vi "createTcpServer.vi"(8 "error in (no error)":errorcluster, 11 "FactoryTcpServer in":refnum<class "FactoryTcpServer.lvclass">) -> (0 "error out":errorcluster, 2 "TcpServer out":refnum<class "TcpServer.lvclass">, 3 "FactoryTcpServer out":refnum<class "FactoryTcpServer.lvclass">)   [LabVIEW 2018, in "FactoryTcpServer.lvclass"]
doc: "Create a new instance of TcpServer class."
uses:
  FactoryTcpServer.lvclass
  TcpServer/TcpServer.lvclass
  TcpServerBase/TcpServerBase.lvclass
  TcpServerCmd/TcpServerCmd.lvclass
  home/pcortes/Documents/github/ts_labview_tcp_json/src/TcpServerBase/TcpServerBase.lvclass
  TcpServerTel/TcpServerTel.lvclass
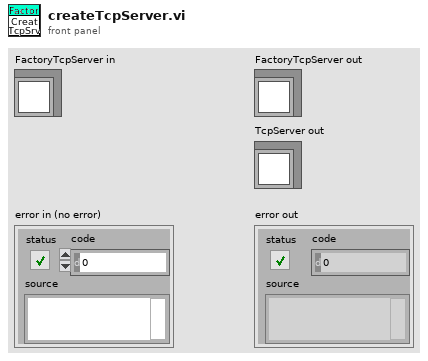
[diagram p1: front panel]
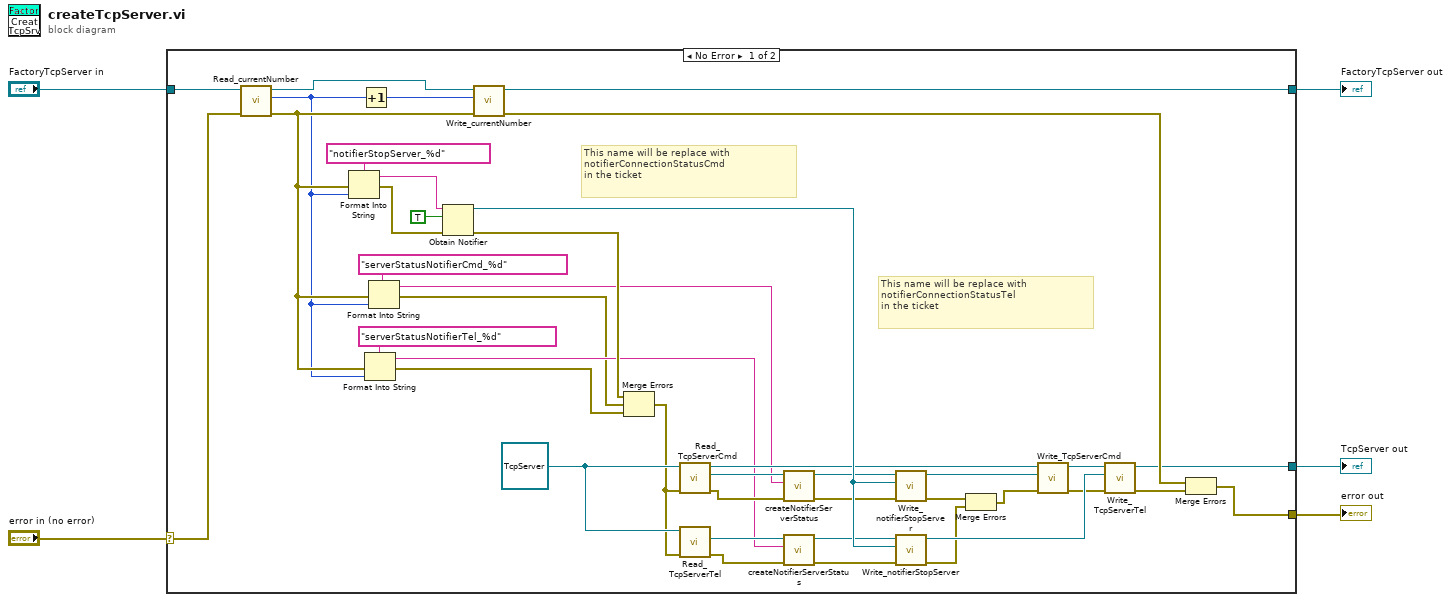
[diagram p0: block diagram]
diagram:
  n1 = case shown="No Error" "error in (no error)" {
    selector: "error in (no error)" -> [w45 w48]
    tunnel: "FactoryTcpServer in" -> [w46 w47]
    tunnel: [w25 w48] -> w3
    tunnel: [w41 w47] -> w2
    tunnel: [w30 _] -> w1
    frame No Error {
      w38 = refnum<class "TcpServer.lvclass"> refnum ("TcpServer.lvclass")
      # "This name will be replace with \nnotifierConnectionStatusTel\nin the ticket"
      # "This name will be replace with \nnotifierConnectionStatusCmd \nin the ticket"
      n2 = call "Read_currentNumber.vi"("error in (no error)"=w45, "FactoryTcpServer in"=w46) -> ("error out"=w20:errorcluster, "currentNumber"=w19:i32, "FactoryTcpServer out"=w42:refnum<class "FactoryTcpServer.lvclass">)  [unwired: 7 in]
      n3 = Format Into String(format string="notifierStopServer_%d", error in=w20, w19) -> (resulting string=w39:string, error out=w23:errorcluster)  [unwired: 1 in]
      n4 = Increment(x=w19) -> (x+1=w44:i32)
      n5 = Format Into String(format string="serverStatusNotifierTel_%d", error in=w20, w19) -> (resulting string=w8:string, error out=w6:errorcluster)  [unwired: 1 in]
      n6 = Format Into String(format string="serverStatusNotifierCmd_%d", error in=w20, w19) -> (resulting string=w10:string, error out=w7:errorcluster)  [unwired: 1 in]
      n7 = Obtain Notifier(name (unnamed)=w39, notification data type=TRUE, error in (no error)=w23) -> (notifier out=w36:refnum<notifier>, error out=w11:errorcluster)  [unwired: 1 in, 1 out]
      n8 = call "Write_currentNumber.vi"("error in (no error)"=w20, "currentNumber"=w44, "FactoryTcpServer in"=w42) -> ("error out"=w43:errorcluster, "FactoryTcpServer out"=w41:refnum<class "FactoryTcpServer.lvclass">)  [unwired: 7 in]
      n9 = Merge Errors(w11, w7, w6) -> (w12:errorcluster)
      n10 = call "Read_TcpServerCmd.vi"("error in (no error)"=w12, "TcpServer in"=w38) -> ("error out"=w9:errorcluster, "TcpServerCmd.lvclass"=w18:refnum<class "TcpServerCmd.lvclass">, "TcpServer out"=w34:refnum<class "TcpServer.lvclass">)  [unwired: 7 in]
      n11 = call "Read_TcpServerTel.vi"("error in (no error)"=w12, "TcpServer in"=w38) -> ("error out"=w29:errorcluster, "TcpServerTel.lvclass"=w15:refnum<class "TcpServerTel.lvclass">)  [unwired: 7 in, 1 out]
      n12 = call "createNotifierServerStatus.vi"("error in (no error)"=w9, "notifierName (unnamed)"=w10, "tcpServerBase in"=w18) -> ("error out"=w13:errorcluster, "tcpServerBase out"=w17:refnum<class "TcpServerCmd.lvclass">)  [unwired: 7 in]
      n13 = call "createNotifierServerStatus.vi"("error in (no error)"=w29, "notifierName (unnamed)"=w8, "tcpServerBase in"=w15) -> ("error out"=w16:errorcluster, "tcpServerBase out"=w14:refnum<class "TcpServerTel.lvclass">)  [unwired: 7 in]
      n14 = call "Write_notifierStopServer.vi"("error in (no error)"=w13, "notifierStopServer"=w36, "TcpServerBase in"=w17) -> ("error out"=w28:errorcluster, "TcpServerBase out"=w35:refnum<class "TcpServerCmd.lvclass">)  [unwired: 7 in]
      n15 = call "Write_notifierStopServer.vi"("error in (no error)"=w16, "notifierStopServer"=w36, "TcpServerBase in"=w14) -> ("error out"=w27:errorcluster, "TcpServerBase out"=w33:refnum<class "TcpServerTel.lvclass">)  [unwired: 7 in]
      n16 = Merge Errors(w28, w27) -> (w26:errorcluster)
      n17 = call "Write_TcpServerCmd.vi"("error in (no error)"=w26, "TcpServerCmd.lvclass"=w35, "TcpServer in"=w34) -> ("error out"=w32:errorcluster, "TcpServer out"=w31:refnum<class "TcpServer.lvclass">)  [unwired: 7 in]
      n18 = call "Write_TcpServerTel.vi"("error in (no error)"=w32, "TcpServerTel.lvclass"=w33, "TcpServer in"=w31) -> ("error out"=w24:errorcluster, "TcpServer out"=w30:refnum<class "TcpServer.lvclass">)  [unwired: 7 in]
      n19 = Merge Errors(w43, w24) -> (w25:errorcluster)
    }
    frame Error {
    }
  }
  "error out" <- w3
  "FactoryTcpServer out" <- w2
  "TcpServer out" <- w1
